vi "8HP_AVmod_Convert serial string to Eng vals.vi"(0 "Serial buffer string (excluding FrameChars and MsgLen word)":string) -> (11 "All vals":sgl[](array[numeric]), 12 "Pressures":sgl[][](graph), 13 "Gyration vector (deg / s)":sgl[](array[numeric]), 14 "Atmospheric pressure (mbar)":sgl, 15 "External thermistor 0 temperature (deg C)":sgl, 16 "External thermistor 1 temperature (deg C)":sgl, 17 "Env. sensor die temperature (deg C)":sgl, 18 "Relative humidity (%)":sgl, 19 "Acceleration vector (g)":sgl[](array[numeric]))   [LabVIEW 2018]
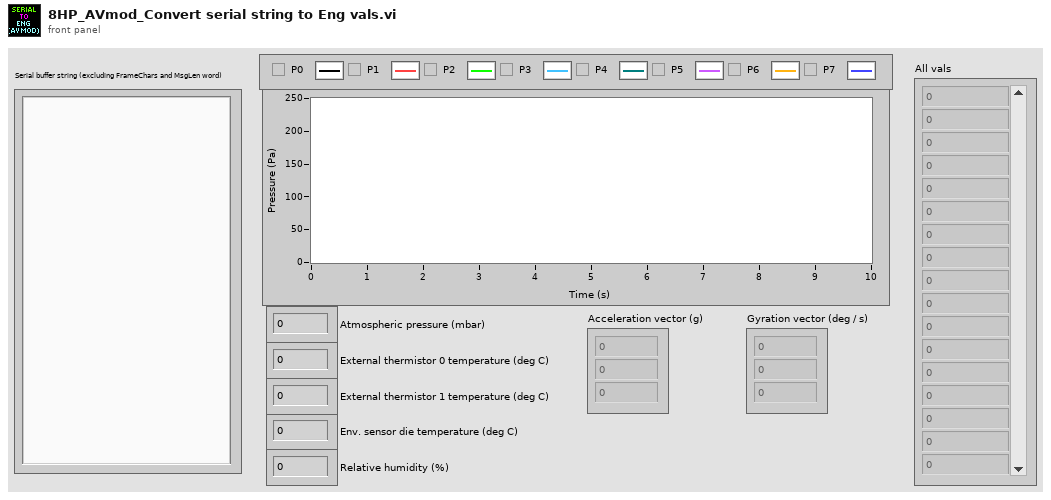
[diagram p1: front panel]
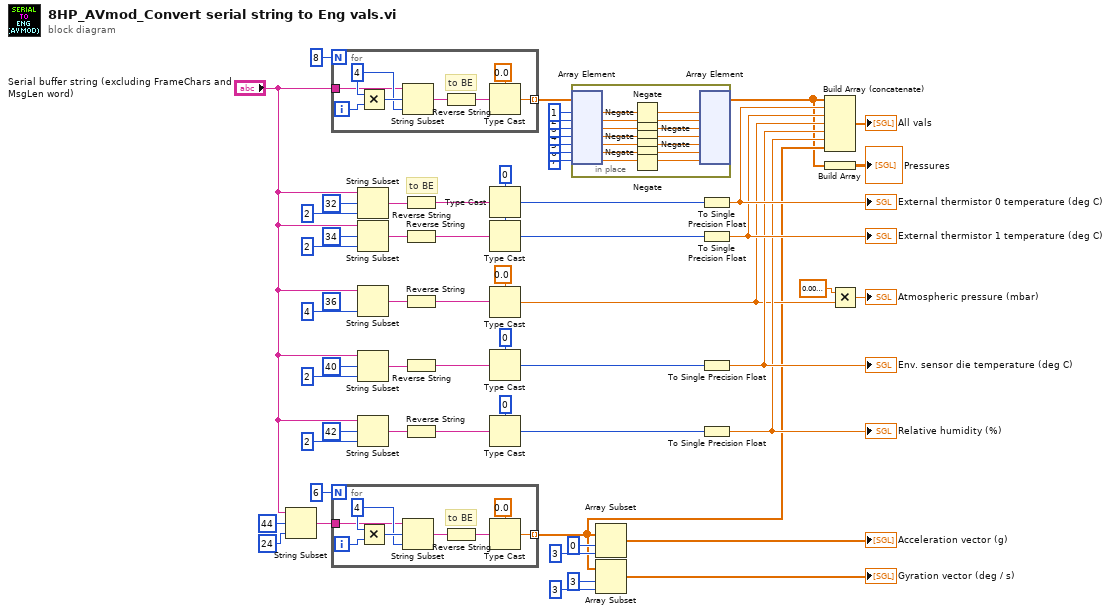
[diagram p0: block diagram]
diagram:
  w35 = i16 0 ("byte count")
  (unwired) 36 ("offset (0)")
  # "to BE"
  n1 = String Subset(string="Serial buffer string (excluding FrameChars and MsgLen word)", offset (0)=44, length (rest)=24 ("length (rest)")) -> (substring=w22:string)
  n2 = for {
    N: 8 -> [_]
    tunnel: [w60] -> w55 mode=indexing
    tunnel: "Serial buffer string (excluding FrameChars and MsgLen word)" -> [w59]
    i -> [w66]
    w64 = 4 ("x")
    # "to BE"
    n3 = Multiply(x=w64, y=w66) -> (x*y=w65:i32)
    n4 = String Subset(string=w59, offset (0)=w65, length (rest)=w64) -> (substring=w63:string)
    n5 = Reverse String(1:w63) -> (0:w62:string)
    n6 = Type Cast(type=sgl 0.0 ("byte count"), x=w62) -> (*(type *) &x=w60:sgl)
  }
  n7 = for {
    N: 6 -> [_]
    tunnel: [w68] -> w3 mode=indexing
    tunnel: w22 -> [w67]
    i -> [w74]
    w72 = 4 ("x")
    # "to BE"
    n8 = Multiply(x=w72, y=w74) -> (x*y=w73:i32)
    n9 = String Subset(string=w67, offset (0)=w73, length (rest)=w72) -> (substring=w71:string)
    n10 = Reverse String(1:w71) -> (0:w70:string)
    n11 = Type Cast(type=sgl 0.0 ("byte count"), x=w70) -> (*(type *) &x=w68:sgl)
  }
  n12 = String Subset(string="Serial buffer string (excluding FrameChars and MsgLen word)", offset (0)=32, length (rest)=2 ("length (rest)")) -> (substring=w43:string)
  n13 = String Subset(string="Serial buffer string (excluding FrameChars and MsgLen word)", offset (0)=34, length (rest)=2 ("length (rest)")) -> (substring=w42:string)
  n14 = String Subset(string="Serial buffer string (excluding FrameChars and MsgLen word)", length (rest)=4 ("length (rest)")) -> (substring=w40:string)  [unwired: 1 in]
  n15 = String Subset(string="Serial buffer string (excluding FrameChars and MsgLen word)", offset (0)=40, length (rest)=2 ("length (rest)")) -> (substring=w30:string)
  n16 = String Subset(string="Serial buffer string (excluding FrameChars and MsgLen word)", offset (0)=42, length (rest)=2 ("length (rest)")) -> (substring=w31:string)
  n17 = Reverse String(1:w43) -> (0:w36:string)
  n18 = Reverse String(1:w42) -> (0:w37:string)
  n19 = Reverse String(1:w40) -> (0:w38:string)
  n20 = Reverse String(1:w30) -> (0:w33:string)
  n21 = Reverse String(1:w31) -> (0:w32:string)
  n22 = Type Cast(type=w35, x=w36) -> (*(type *) &x=w15:i16)
  n23 = Type Cast(type=w35, x=w37) -> (*(type *) &x=w14:i16)
  n24 = Type Cast(type=sgl 0.0 ("byte count"), x=w38) -> (*(type *) &x=w4:sgl)
  n25 = Type Cast(type=i16 0 ("byte count"), x=w33) -> (*(type *) &x=w13:i16)
  n26 = Type Cast(type=u16 0 ("byte count"), x=w32) -> (*(type *) &x=w12:u16)
  n27 = in-place {
    n28 = in-place-array #1(w55, 1, 2, 3, 4, 5, 6, 7) -> (w88:sgl, w87:sgl, w84:sgl, w83:sgl, w82:sgl, w76:sgl, w81:sgl)
    n29 = Negate(x=w88) -> (-x=w86:sgl)
    n30 = Negate(x=w87) -> (-x=w85:sgl)
    n31 = Negate(x=w84) -> (-x=w80:sgl)
    n32 = Negate(x=w83) -> (-x=w79:sgl)
    n33 = Negate(x=w82) -> (-x=w78:sgl)
    n34 = Negate(x=w76) -> (-x=w75:sgl)
    n35 = Negate(x=w81) -> (-x=w77:sgl)
    n36 = in-place-array #1(w86, w85, w80, w79, w78, w75, w77) -> (w1:sgl[])  [unwired: 7 out]
  }
  n37 = Array Subset(array=w3, index=0, length=3) -> (→"Acceleration vector (g)":sgl[])
  n38 = Array Subset(array=w3, index=3, length=3) -> (→"Gyration vector (deg / s)":sgl[])
  n39 = To Single Precision Float(number=w15) -> (single precision float=w11:sgl)
  "External thermistor 0 temperature (deg C)" <- w11
  n40 = To Single Precision Float(number=w14) -> (single precision float=w10:sgl)
  "External thermistor 1 temperature (deg C)" <- w10
  n41 = To Single Precision Float(number=w13) -> (single precision float=w8:sgl)
  "Env. sensor die temperature (deg C)" <- w8
  n42 = To Single Precision Float(number=w12) -> (single precision float=w7:sgl)
  "Relative humidity (%)" <- w7
  n43 = Build Array (concatenate)(w1, w11, w10, w4, w8, w7, w3) -> (→"All vals":sgl[])
  n44 = Build Array(w1) -> (→"Pressures":sgl[][])
  n45 = Multiply(x=sgl 0.01, y=w4) -> (x*y=→"Atmospheric pressure (mbar)":sgl)
